vi "getValores.vi"(8 "error in (no error)":errorcluster, 9 "verificação":string, 10 "enviar código":string, 11 "VISA Refnum in":refnum<visa-resource-name>) -> (0 "error out":errorcluster, 2 "number":i32, 3 "VISA Refnum out":refnum<visa-resource-name>)   [LabVIEW 2018]
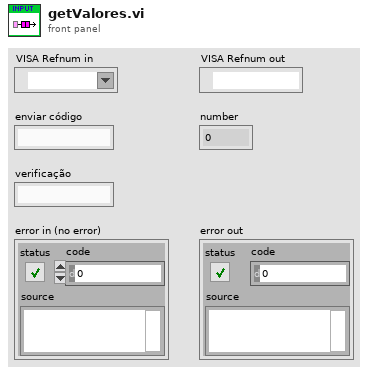
[diagram p1: front panel]
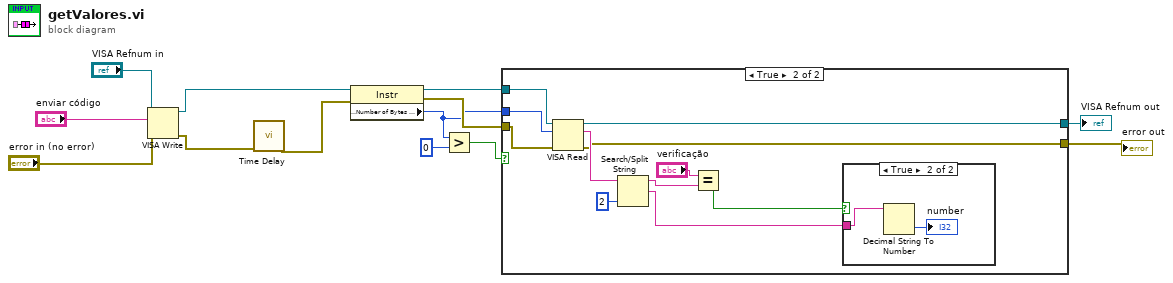
[diagram p0: block diagram]
diagram:
  n1 = VISA Write(VISA resource name="VISA Refnum in", write buffer="enviar código", error in (no error)="error in (no error)") -> (VISA resource name out=w10:refnum<visa-resource-name>, error out=w12:errorcluster)  [unwired: 1 out]
  n2 = call "Time Delay"("error in (no error)"=w12) -> ("error out"=w11:errorcluster)  [unwired: 10 in]
  n3 = property class="Instr"(reference=w10, error in=w11) -> (reference out=w7:refnum<visa-resource-name>, error out=w6:errorcluster, "Serial Settings:Number of Bytes at Serial Port"=w5:u32)
  n4 = Greater?(x=w5, y=u32 0) -> (0:w8:bool)
  n5 = case shown="True" w8 {
    tunnel: w7 -> [w15 w26]
    tunnel: w6 -> [w14 w25]
    tunnel: w5 -> [_ w24]
    tunnel: [w15 w18] -> w2
    tunnel: [w14 w17] -> w1
    frame False {
    }
    frame True {
      n6 = VISA Read(VISA resource name=w26, byte count=w24, error in (no error)=w25) -> (VISA resource name out=w18:refnum<visa-resource-name>, read buffer=w22:string, error out=w17:errorcluster)  [unwired: 1 out]
      n7 = Search/Split String(string=w22, offset (0)=2) -> (substring before match=w21:string, match + rest of string=w19:string)  [unwired: 1 in, 1 out]
      n8 = Equal?(x="verificação", y=w21) -> (x = y?=w20:bool)
      n9 = case shown="True" w20 {
        tunnel: w19 -> [_ w28]
        frame False {
        }
        frame True {
          n10 = Decimal String To Number(string=w28) -> (number=→"number":i32)  [unwired: 2 in, 1 out]
        }
      }
    }
  }
  "VISA Refnum out" <- w2
  "error out" <- w1
